vi "Read Onboard Temperature.vi"(8 "error in (no error)":errorcluster, 11 "VISA resource name in":refnum<visa-resource-name>) -> (0 "error out":errorcluster, 2 "Temp degC":dbl, 3 "VISA resource name":refnum<visa-resource-name>)   [LabVIEW 2020, in "CTI-Visa-Pico.lvlib"]
doc: "Reads the onboard temperature sensor in Degrees Celcius. This reading is low resolution and not very accurate."
uses:
  CTI-Visa-Pico.lvlib
  CTI-Visa/CTI-Visa.lvlib
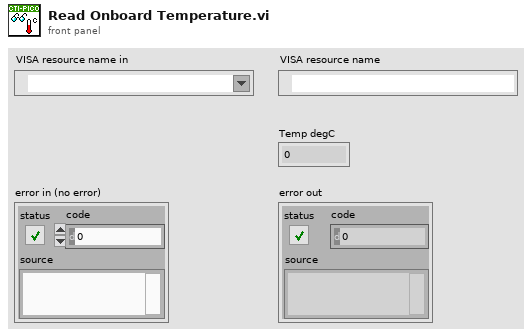
[diagram p1: front panel]
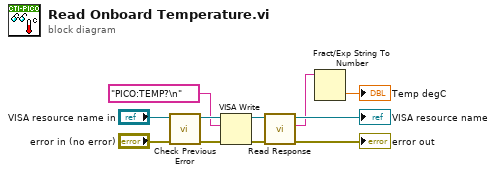
[diagram p0: block diagram]
diagram:
  n1 = call "Check Previous Error.vi"("error in (no error)"="error in (no error)", "VISA resource name in"="VISA resource name in") -> ("error out"=w8:errorcluster, "VISA resource name"=w9:refnum<visa-resource-name>)  [unwired: 8 in]
  n2 = VISA Write(VISA resource name=w9, write buffer="PICO:TEMP?\n" ("format string"), error in (no error)=w8) -> (VISA resource name out=w10:refnum<visa-resource-name>, error out=w11:errorcluster)  [unwired: 1 out]
  n3 = call "Read Response.vi"("error in (no error)"=w11, "VISA resource name in"=w10) -> ("error out"=→"error out":errorcluster, "Response"=w3:string, "VISA resource name"=→"VISA resource name":refnum<visa-resource-name>)  [unwired: 7 in]
  n4 = Fract/Exp String To Number(string=w3) -> (number=→"Temp degC":dbl)  [unwired: 3 in, 1 out]
